vi "py.create.Pitch.vi"(8 "error in (no error)":errorcluster, 11 "Parameters":variant) -> (0 "error out":errorcluster, 3 "bytes":u8[](array[numeric]) format="%.0x")   [LabVIEW 2022 SP3]
uses:
  AddOrder/AddOrderLong.Parameters.ctl
  Time/Time.Parameters.ctl
  OrderExecuted/OrderExecuted.Parameters.ctl
  ReduceSize/ReduceSizeLong.Parameters.ctl
  ReduceSize/ReduceSizeShort.Parameters.ctl
  ModifyOrder/ModifyOrderLong.Parameters.ctl
  ModifyOrder/ModifyOrderShort.Parameters.ctl
  DeleteOrder/DeleteOrder.Parameters.ctl
  Trade/TradeLong.Parameters.ctl
  Trade/TradeShort.Parameters.ctl
  Trade/TradeExpanded.Parameters.ctl
  AddOrder/AddOrderShort.Parameters.ctl
  AddOrder/AddOrderExpanded.Parameters.ctl
  OrderExecuted/OrderExecutedAtPriceSize.Parameters.ctl
  <vilib>/Utility/Data Type/NI_Data Type.lvlib
  AddOrder/AddOrderLong.lvclass
  Time/Time.lvclass
  OrderExecuted/OrderExecuted.lvclass
  ReduceSize/ReduceSizeLong.lvclass
  ReduceSize/ReduceSizeShort.lvclass
  ModifyOrder/ModifyOrderLong.lvclass
  ModifyOrder/ModifyOrderShort.lvclass
  DeleteOrder/DeleteOrder.lvclass
  Trade/TradeLong.lvclass
  Trade/TradeShort.lvclass
  Trade/TradeExpanded.lvclass
  AddOrder/AddOrderShort.lvclass
  AddOrder/AddOrderExpanded.lvclass
  OrderExecuted/OrderExecutedAtPriceSize.lvclass
panel:
  out "name":string
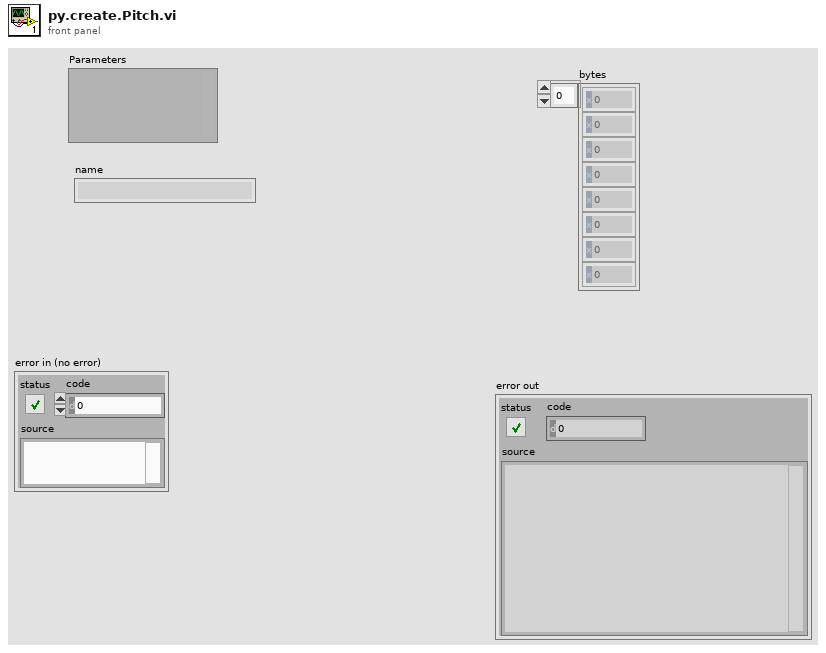
[diagram p1: front panel]
types:
  T1 = typedef "AddOrderLong.lvclass/AddOrderLong.Parameters.ctl" = cluster{"Time Offset":u32, "Order Id":string, "Quantity":u32, "Symbol":string, "Side Indicator":string, "Price":dbl}
  T2 = typedef "Time.lvclass/Time.Parameters.ctl" = cluster{"Time":u32}
  T3 = typedef "OrderExecuted.lvclass/OrderExecuted.Parameters.ctl" = cluster{"Time Offset":u32, "Order Id":string, "Executed Quantity":u32, "Execution Id":string}
  T4 = typedef "ReduceSizeLong.lvclass/ReduceSizeLong.Parameters.ctl" = cluster{"Time Offset":u32, "Order Id":string, "Canceled Quantity":u32}
  T5 = typedef "ReduceSizeShort.lvclass/ReduceSizeShort.Parameters.ctl" = cluster{"Time Offset":u32, "Order Id":string, "Canceled Quantity":u16}
  T6 = typedef "ModifyOrderLong.lvclass/ModifyOrderLong.Parameters.ctl" = cluster{"Time Offset":u32, "Order Id":string, "Quantity":u32, "Price":dbl, "Modify Flags":u8}
  T7 = typedef "ModifyOrderShort.lvclass/ModifyOrderShort.Parameters.ctl" = cluster{"Time Offset":u32, "Order Id":string, "Quantity":u32, "Price":u16, "Modify Flags":u8}
  T8 = typedef "DeleteOrder.lvclass/DeleteOrder.Parameters.ctl" = cluster{"Time Offset":u32, "Order Id":string}
  T9 = typedef "TradeLong.lvclass/TradeLong.Parameters.ctl" = cluster{"Time Offset":u32, "Order Id":string, "Execution Id":string, "Quantity":u32, "Price":dbl, "Side Indicator":string, "Symbol":string}
  T10 = typedef "TradeShort.lvclass/TradeShort.Parameters.ctl" = cluster{"Time Offset":u32, "Order Id":string, "Execution Id":string, "Quantity":u32, "Price":dbl, "Side Indicator":string, "Symbol":string}
  T11 = typedef "TradeExpanded.lvclass/TradeExpanded.Parameters.ctl" = cluster{"Time Offset":u32, "Order Id":string, "Side Indicator":string, "Quantity":u32, "Symbol":string, "Price":dbl, "Execution Id":string}
  T12 = typedef "AddOrderShort.lvclass/AddOrderShort.Parameters.ctl" = cluster{"Time Offset":u32, "Order Id":string, "Quantity":u32, "Symbol":string, "Side Indicator":string, "Price":dbl}
  T13 = typedef "AddOrderExpanded.lvclass/AddOrderExpanded.Parameters.ctl" = cluster{"Time Offset":u32, "Order Id":string, "Quantity":u32, "Symbol":string, "Side Indicator":string, "Price":dbl, "Participant Id":string, "Customer Indicator":string}
  T14 = typedef "OrderExecutedAtPriceSize.lvclass/OrderExecutedAtPriceSize.Parameters.ctl" = cluster{"Time Offset":u32, "Order Id":string, "Executed Quantity":u32, "Execution Id":string, "Remaining Quantity":u32, "Price":dbl}
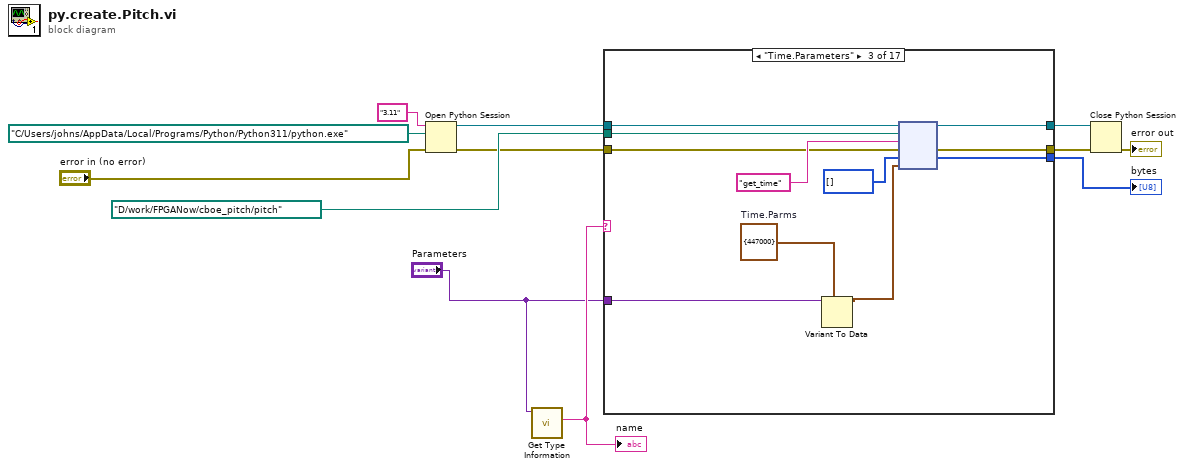
[diagram p0: block diagram]
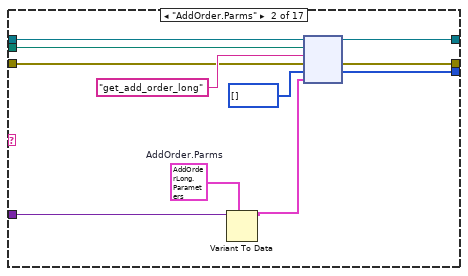
[diagram p3: hidden frame]
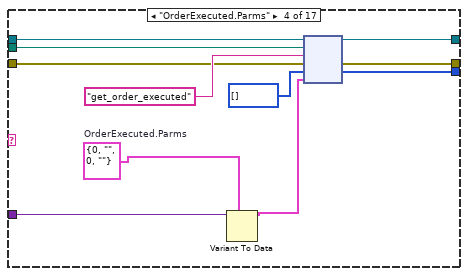
[diagram p4: hidden frame]
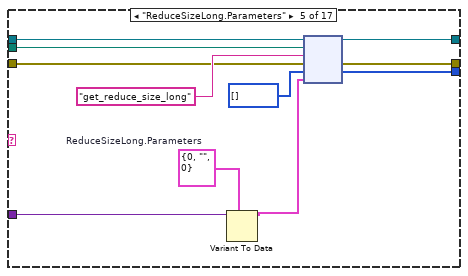
[diagram p5: hidden frame]
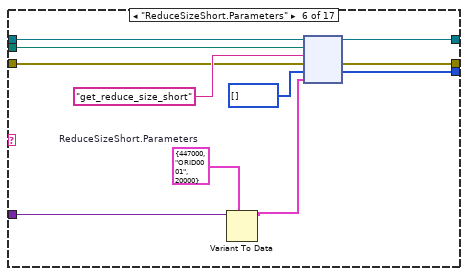
[diagram p6: hidden frame]
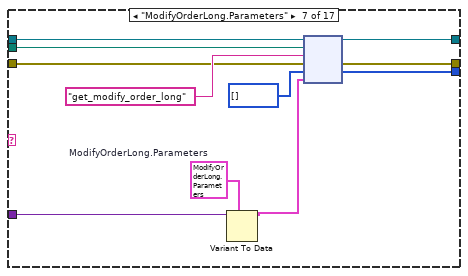
[diagram p7: hidden frame]
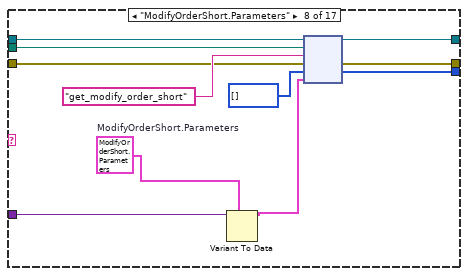
[diagram p8: hidden frame]
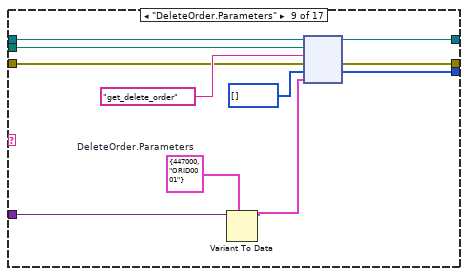
[diagram p9: hidden frame]
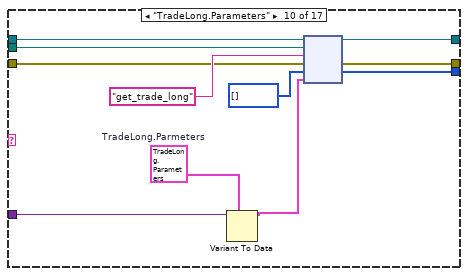
[diagram p10: hidden frame]
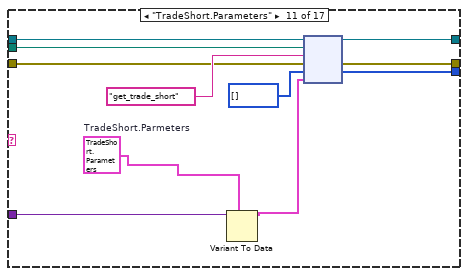
[diagram p11: hidden frame]
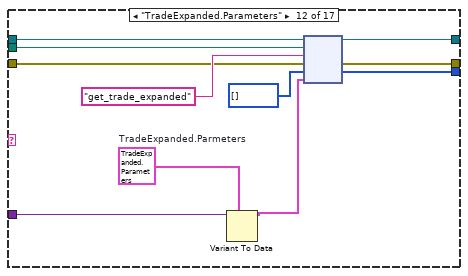
[diagram p12: hidden frame]
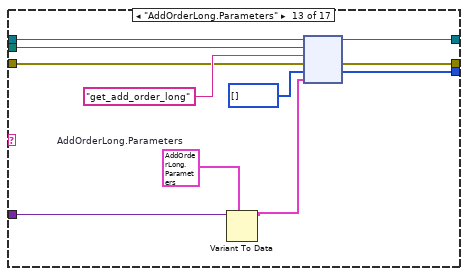
[diagram p13: hidden frame]
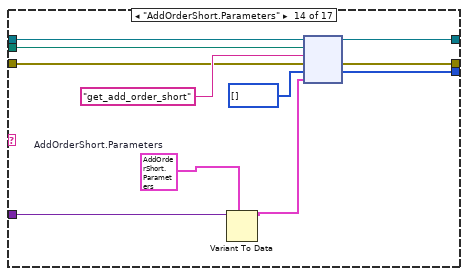
[diagram p14: hidden frame]
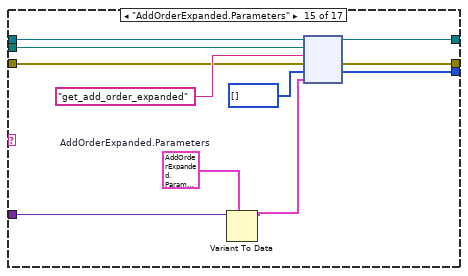
[diagram p15: hidden frame]
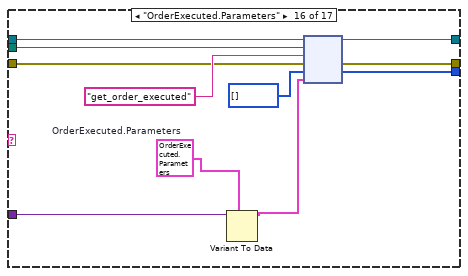
[diagram p16: hidden frame]
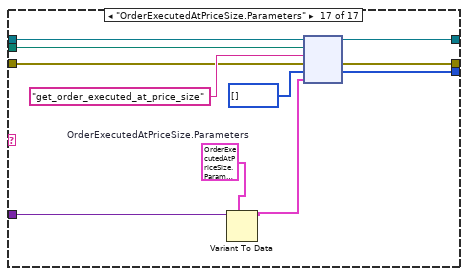
[diagram p17: hidden frame]
diagram:
  n1 = Open Python Session(python version="3.11" ("Python version"), python path=path "C:/Users/johns/AppData/Local/Programs/Python/Python311/python.exe" ("Python path"), 3:"error in (no error)") -> (session out=w12:refnum<k35>, error out=w6:errorcluster)
  n2 = call <vilib>:"Get Type Information.vi"("variant"="Parameters") -> ("name"=w2:string)  [unwired: 6 in, 4 out]
  "name" <- w2
  n3 = case shown="\"Time.Parameters\"" w2 {
    tunnel: w12 -> [w14 w25 w36 w47 w58 w69 w80 w91 w102 w113 w124 w135 w146 w157 w168 w179 w190]
    tunnel: [w14 w24 w35 w46 w57 w68 w79 w90 w101 w112 w123 w134 w145 w156 w167 w178 w189] -> w11
    tunnel: path "D:/work/FPGANow/cboe_pitch/pitch" ("module path") -> [_ w23 w34 w45 w56 w67 w78 w89 w100 w111 w122 w133 w144 w155 w166 w177 w188]
    tunnel: [w13 w22 w33 w44 w55 w66 w77 w88 w99 w110 w121 w132 w143 w154 w165 w176 w187] -> w7
    tunnel: w6 -> [w13 w20 w31 w42 w53 w64 w75 w86 w97 w108 w119 w130 w141 w152 w163 w174 w185]
    tunnel: [_ w19 w30 w41 w52 w63 w74 w85 w96 w107 w118 w129 w140 w151 w162 w173 w184] -> w5
    tunnel: "Parameters" -> [_ w17 w28 w39 w50 w61 w72 w83 w94 w105 w116 w127 w138 w149 w160 w171 w182]
    frame "False", Default {
    }
    frame "AddOrder.Parms" {
      w16 = T1 {"Time Offset"=447000, "Order Id"="ORID0001", "Quantity"=20000, "Symbol"="AAPL", "Side Indicator"="B", "Price"=0.905}  # AddOrder.Parms
      n4 = Variant To Data(type=w16, Variant=w17) -> (data=w15:T1)  [unwired: 1 in, 1 out]
      n5 = node(w25, w23, "get_add_order_long" ("function name"), w20, u8[] [], w15) -> (w24:refnum<k35>, w22:errorcluster, w19:u8[])  [unwired: 1 in, 2 out]
    }
    frame "Time.Parameters" {
      w26 = T2 {"Time"=447000}  # Time.Parms
      n6 = Variant To Data(type=w26, Variant=w28) -> (data=w27:T2)  [unwired: 1 in, 1 out]
      n7 = node(w36, w34, "get_time" ("function name"), w31, u8[] [], w27) -> (w35:refnum<k35>, w33:errorcluster, w30:u8[])  [unwired: 1 in, 2 out]
    }
    frame "OrderExecuted.Parms" {
      w37 = T3 {"Time Offset"=0, "Order Id"="", "Executed Quantity"=0, "Execution Id"=""}  # OrderExecuted.Parms
      n8 = Variant To Data(type=w37, Variant=w39) -> (data=w38:T3)  [unwired: 1 in, 1 out]
      n9 = node(w47, w45, "get_order_executed" ("function name"), w42, u8[] [], w38) -> (w46:refnum<k35>, w44:errorcluster, w41:u8[])  [unwired: 1 in, 2 out]
    }
    frame "ReduceSizeLong.Parameters" {
      w48 = T4 {"Time Offset"=0, "Order Id"="", "Canceled Quantity"=0}  # ReduceSizeLong.Parameters
      n10 = Variant To Data(type=w48, Variant=w50) -> (data=w49:T4)  [unwired: 1 in, 1 out]
      n11 = node(w58, w56, "get_reduce_size_long" ("function name"), w53, u8[] [], w49) -> (w57:refnum<k35>, w55:errorcluster, w52:u8[])  [unwired: 1 in, 2 out]
    }
    frame "ReduceSizeShort.Parameters" {
      w59 = T5 {"Time Offset"=447000, "Order Id"="ORID0001", "Canceled Quantity"=20000}  # ReduceSizeShort.Parameters
      n12 = Variant To Data(type=w59, Variant=w61) -> (data=w60:T5)  [unwired: 1 in, 1 out]
      n13 = node(w69, w67, "get_reduce_size_short" ("function name"), w64, u8[] [], w60) -> (w68:refnum<k35>, w66:errorcluster, w63:u8[])  [unwired: 1 in, 2 out]
    }
    frame "ModifyOrderLong.Parameters" {
      w70 = T6 {"Time Offset"=447000, "Order Id"="ORID0001", "Quantity"=20000, "Price"=0.905, "Modify Flags"=1}  # ModifyOrderLong.Parameters
      n14 = Variant To Data(type=w70, Variant=w72) -> (data=w71:T6)  [unwired: 1 in, 1 out]
      n15 = node(w80, w78, "get_modify_order_long" ("function name"), w75, u8[] [], w71) -> (w79:refnum<k35>, w77:errorcluster, w74:u8[])  [unwired: 1 in, 2 out]
    }
    frame "ModifyOrderShort.Parameters" {
      w81 = T7 {"Time Offset"=447000, "Order Id"="ORID0001", "Quantity"=20000, "Price"=1, "Modify Flags"=1}  # ModifyOrderShort.Parameters
      n16 = Variant To Data(type=w81, Variant=w83) -> (data=w82:T7)  [unwired: 1 in, 1 out]
      n17 = node(w91, w89, "get_modify_order_short" ("function name"), w86, u8[] [], w82) -> (w90:refnum<k35>, w88:errorcluster, w85:u8[])  [unwired: 1 in, 2 out]
    }
    frame "DeleteOrder.Parameters" {
      w92 = T8 {"Time Offset"=447000, "Order Id"="ORID0001"}  # DeleteOrder.Parameters
      n18 = Variant To Data(type=w92, Variant=w94) -> (data=w93:T8)  [unwired: 1 in, 1 out]
      n19 = node(w102, w100, "get_delete_order" ("function name"), w97, u8[] [], w93) -> (w101:refnum<k35>, w99:errorcluster, w96:u8[])  [unwired: 1 in, 2 out]
    }
    frame "TradeLong.Parameters" {
      w103 = T9 {"Time Offset"=447000, "Order Id"="ORID0001", "Execution Id"="EXE_ID_1", "Quantity"=20000, "Price"=0.905, "Side Indicator"="B", "Symbol"="AAPL"}  # TradeLong.Parmeters
      n20 = Variant To Data(type=w103, Variant=w105) -> (data=w104:T9)  [unwired: 1 in, 1 out]
      n21 = node(w113, w111, "get_trade_long" ("function name"), w108, u8[] [], w104) -> (w112:refnum<k35>, w110:errorcluster, w107:u8[])  [unwired: 1 in, 2 out]
    }
    frame "TradeShort.Parameters" {
      w114 = T10 {"Time Offset"=447000, "Order Id"="ORID0001", "Execution Id"="EXE_ID_1", "Quantity"=20000, "Price"=0.905, "Side Indicator"="B", "Symbol"="AAPL"}  # TradeShort.Parmeters
      n22 = Variant To Data(type=w114, Variant=w116) -> (data=w115:T10)  [unwired: 1 in, 1 out]
      n23 = node(w124, w122, "get_trade_short" ("function name"), w119, u8[] [], w115) -> (w123:refnum<k35>, w121:errorcluster, w118:u8[])  [unwired: 1 in, 2 out]
    }
    frame "TradeExpanded.Parameters" {
      w125 = T11 {"Time Offset"=447000, "Order Id"="ORID0001", "Side Indicator"="B", "Quantity"=20000, "Symbol"="AAPL", "Price"=0.905, "Execution Id"="EXE_ID_1"}  # TradeExpanded.Parmeters
      n24 = Variant To Data(type=w125, Variant=w127) -> (data=w126:T11)  [unwired: 1 in, 1 out]
      n25 = node(w135, w133, "get_trade_expanded" ("function name"), w130, u8[] [], w126) -> (w134:refnum<k35>, w132:errorcluster, w129:u8[])  [unwired: 1 in, 2 out]
    }
    frame "AddOrderLong.Parameters" {
      w136 = T1 {"Time Offset"=447000, "Order Id"="ORID0001", "Quantity"=20000, "Symbol"="AAPL", "Side Indicator"="B", "Price"=0.905}  # AddOrderLong.Parameters
      n26 = Variant To Data(type=w136, Variant=w138) -> (data=w137:T1)  [unwired: 1 in, 1 out]
      n27 = node(w146, w144, "get_add_order_long" ("function name"), w141, u8[] [], w137) -> (w145:refnum<k35>, w143:errorcluster, w140:u8[])  [unwired: 1 in, 2 out]
    }
    frame "AddOrderShort.Parameters" {
      w147 = T12 {"Time Offset"=447000, "Order Id"="ORID0001", "Quantity"=20000, "Symbol"="AAPL", "Side Indicator"="B", "Price"=0.905}  # AddOrderShort.Parameters
      n28 = Variant To Data(type=w147, Variant=w149) -> (data=w148:T12)  [unwired: 1 in, 1 out]
      n29 = node(w157, w155, "get_add_order_short" ("function name"), w152, u8[] [], w148) -> (w156:refnum<k35>, w154:errorcluster, w151:u8[])  [unwired: 1 in, 2 out]
    }
    frame "AddOrderExpanded.Parameters" {
      w158 = T13 {"Time Offset"=447000, "Order Id"="ORID0001", "Quantity"=20000, "Symbol"="AAPL", "Side Indicator"="B", "Price"=0.905, "Participant Id"="B", "Customer Indicator"="B"}  # AddOrderExpanded.Parameters
      n30 = Variant To Data(type=w158, Variant=w160) -> (data=w159:T13)  [unwired: 1 in, 1 out]
      n31 = node(w168, w166, "get_add_order_expanded" ("function name"), w163, u8[] [], w159) -> (w167:refnum<k35>, w165:errorcluster, w162:u8[])  [unwired: 1 in, 2 out]
    }
    frame "OrderExecuted.Parameters" {
      w169 = T3 {"Time Offset"=447000, "Order Id"="ORID0001", "Executed Quantity"=20000, "Execution Id"="AAPL"}  # OrderExecuted.Parameters
      n32 = Variant To Data(type=w169, Variant=w171) -> (data=w170:T3)  [unwired: 1 in, 1 out]
      n33 = node(w179, w177, "get_order_executed" ("function name"), w174, u8[] [], w170) -> (w178:refnum<k35>, w176:errorcluster, w173:u8[])  [unwired: 1 in, 2 out]
    }
    frame "OrderExecutedAtPriceSize.Parameters" {
      w180 = T14 {"Time Offset"=447000, "Order Id"="ORID0001", "Executed Quantity"=20000, "Execution Id"="AAPL", "Remaining Quantity"=20000, "Price"=0.905}  # OrderExecutedAtPriceSize.Parameters
      n34 = Variant To Data(type=w180, Variant=w182) -> (data=w181:T14)  [unwired: 1 in, 1 out]
      n35 = node(w190, w188, "get_order_executed_at_price_size" ("function name"), w185, u8[] [], w181) -> (w189:refnum<k35>, w187:errorcluster, w184:u8[])  [unwired: 1 in, 2 out]
    }
  }
  "bytes" <- w5
  n36 = Close Python Session(session in=w11, error in=w7) -> (11:→"error out":errorcluster)
